vi "PortsArrayHandler.vi"(2 "Input":i32[](array[numeric])=[2, 2, 2, 2, 2, 2, 2, 2, 2, 2, 2], 3 "Init Input":i32[](array[numeric])=[2, 2, 2, 2, 2, 2, 2, 2, 2, 2, 2], 4 "INPUT PORT states":bool[](array[boolean])) -> (0 "Rezult Input Ports":i32[](array[numeric]), 1 "boolean Ports Array":bool[](array[boolean]))   [LabVIEW 2012]
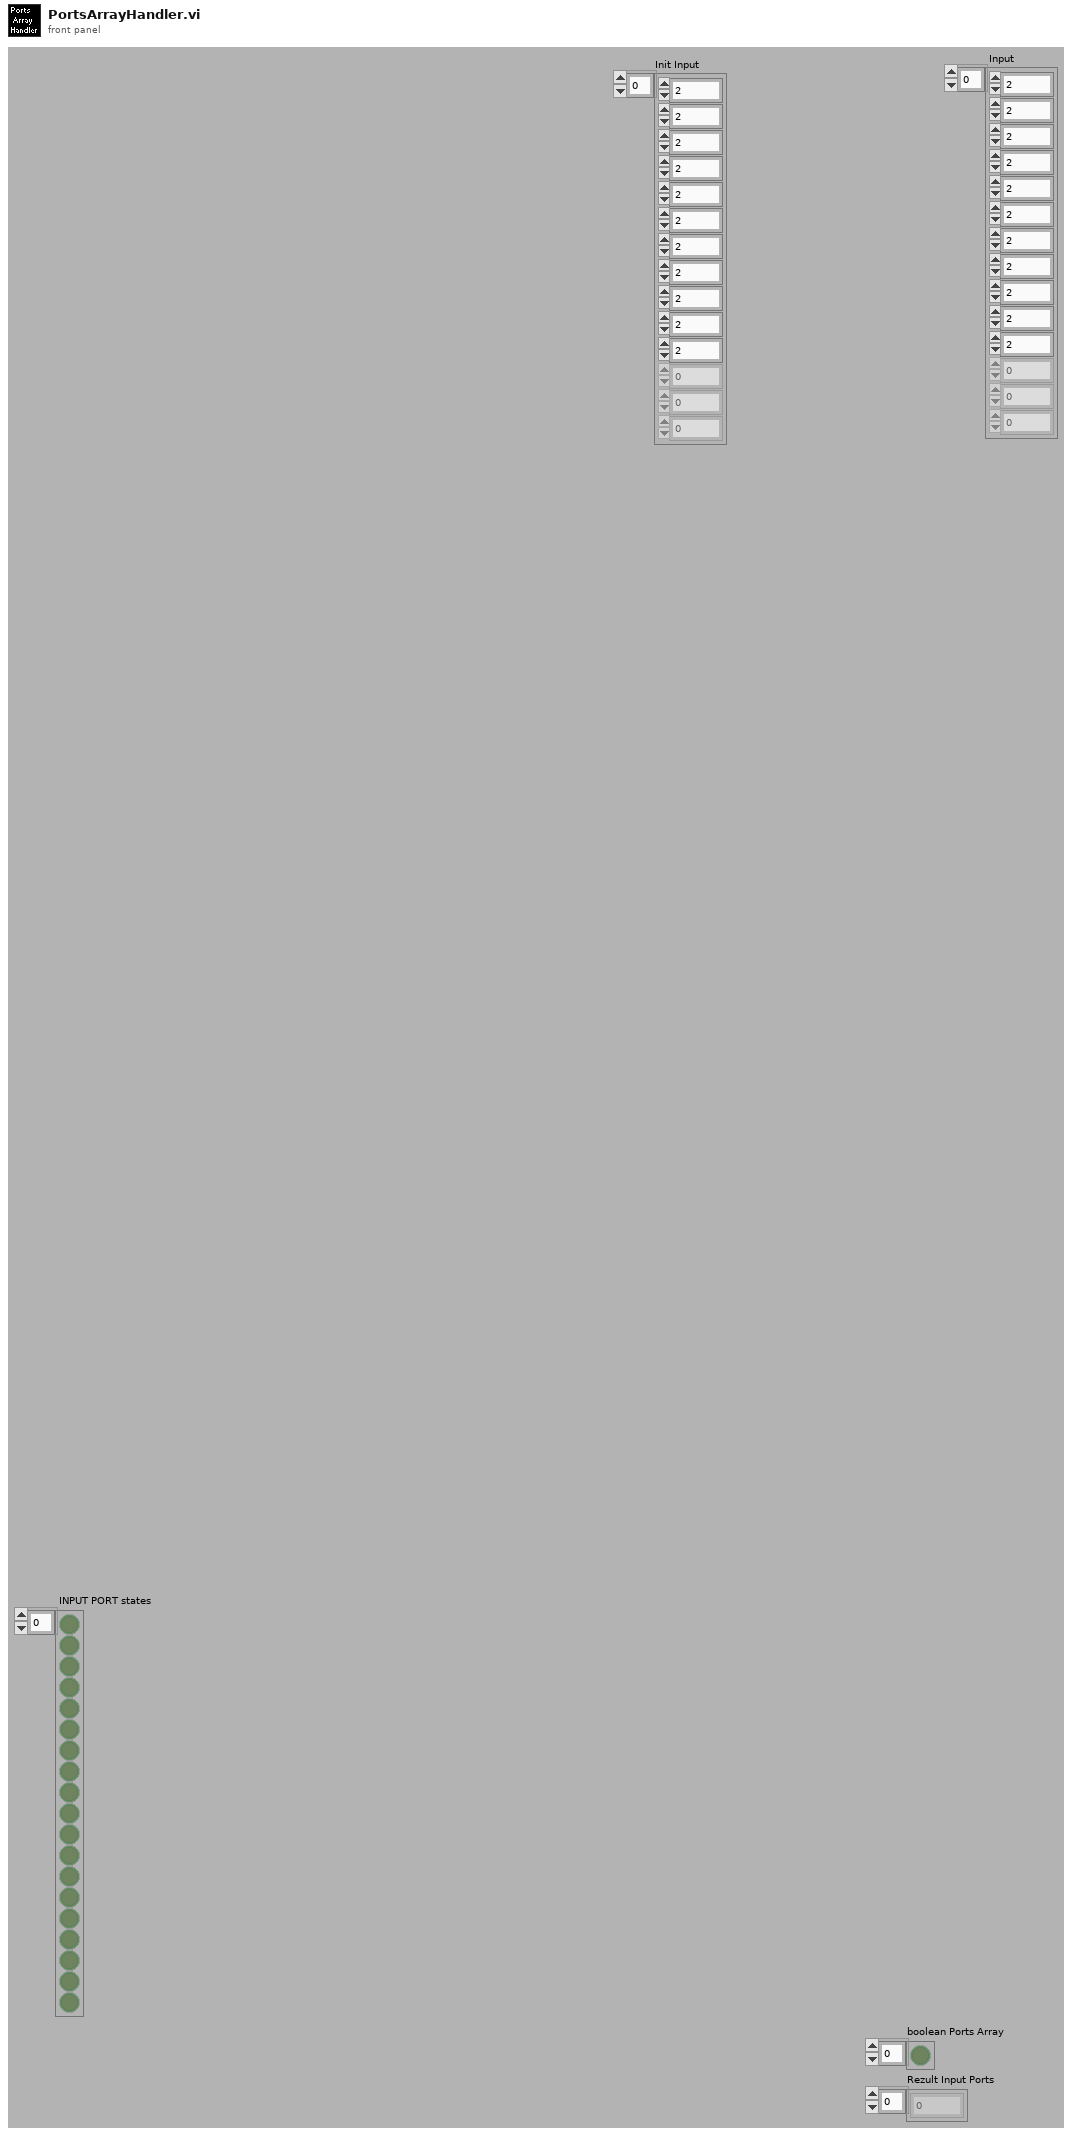
[diagram p1: front panel]
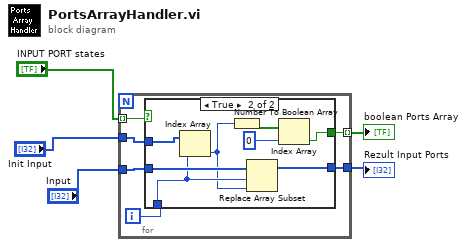
[diagram p0: block diagram]
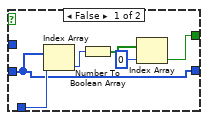
[diagram p2: hidden frame]
diagram:
  n1 = for {
    tunnel: "Input" -> [w9]
    tunnel: "INPUT PORT states" -> [w11] mode=indexing
    tunnel: "Init Input" -> [w7]
    tunnel: [w10] -> w2 mode=indexing
    tunnel: [w6] -> w1
    i -> [w8]
    n2 = case shown="True" w11 {
      tunnel: [w12 w18] -> w10
      tunnel: w9 -> [w16 w24]
      tunnel: w8 -> [w17 w23]
      tunnel: w7 -> [_ w25]
      tunnel: [w16 w22] -> w6
      frame False {
        n3 = Index Array(array=w16, index=w17) -> (element=w13:i32)
        n4 = Number To Boolean Array(number=w13) -> (Boolean array=w14:bool[])
        n5 = Index Array(array=w14, index=0) -> (element=w12:bool)
      }
      frame True {
        n6 = Index Array(array=w25, index=w23) -> (element=w19:i32)
        n7 = Number To Boolean Array(number=w19) -> (Boolean array=w20:bool[])
        n8 = Replace Array Subset(array=w24, new element=w19, index=w23) -> (w22:i32[])
        n9 = Index Array(array=w20, index=0) -> (element=w18:bool)
      }
    }
  }
  "boolean Ports Array" <- w2
  "Rezult Input Ports" <- w1
